vi "Save Raw Data.vi"(1 "data":T1[](array[typedef]) {"time (global)" format="%<%H:%M:%S\n%d/%m/%Y>T"}, 3 "time [ms]":i64, 7 "VI-data Save":T5={"Dateipfad save data"=path "", "file ref"=refnum, "number"=0, "Period [s]"=240, "Fehler (Ausgang)"={"status"=FALSE, "code"=0, "source"=""}}) -> (8 "VI-data Save out":T5={"Dateipfad save data"=path "", "file ref"=refnum, "number"=0, "Period [s]"=240, "Fehler (Ausgang)"={"status"=FALSE, "code"=0, "source"=""}})   [LabVIEW 2010, in "Licor-Steuerung.lvlib"]
uses:
  Licor-Steuerung.lvlib
  VI-data Save.ctl
  control/Licor-Parameter.ctl
  LicorLI7000/conventions/Licor-Source.ctl
  control/Licor-Pump.ctl
  LicorLI7000/conventions/output line.ctl
  LicorLI7000/LicorLI7000.lvlib
panel:
  in  "Licor-parameter":T2={"CO2 ref"=392.0, "CO2 span"=402.0, "H2O ref"=0.0, "H2O span"=0.0, "Zi"=1.2, "Zt"=0.0, "Zm"=0.0, "S"=1.0, "Temp [C]"=50.0, "Pressure [hPa]"=135.0, "Licor-Sources"=["CO2A W", "CO2B W", "H2OA W", "H2OB W", "T C", "T V", "P kPa", "P V", "RH %", "CO2A um/m", "CO2B um/m", "H2OA mm/m", "H2OB mm/m"], "Licor-Pump"="Off", "Zeitstempel"=timestamp(0 s since 1904-01-01)} {"Pressure [hPa]" format="%_5g"; "Temp [C]" format="%.2f"; "CO2 ref" format="%.2f"; "CO2 span" format="%.2g"; "H2O ref" format="%.2g"; "H2O span" format="%.2g"; "Zt" format="%#_4g"}
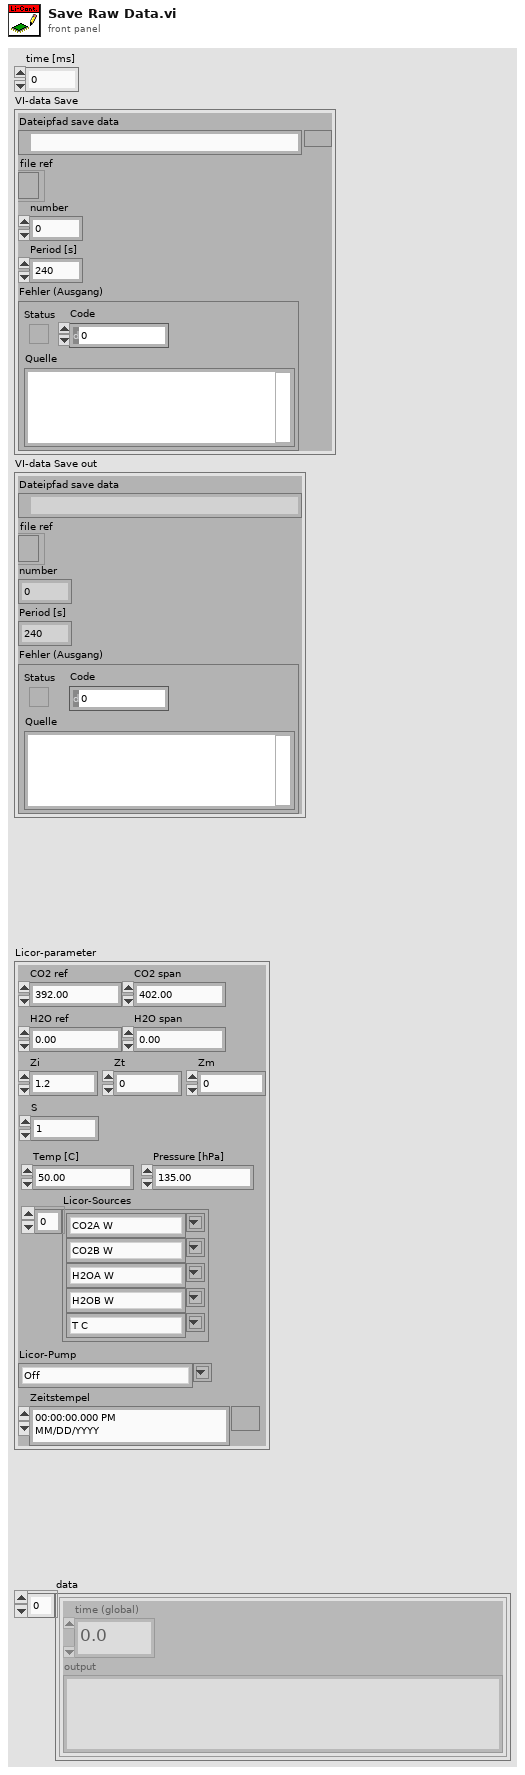
[diagram p1: front panel]
types:
  T1 = typedef "LicorLI7000.lvlib/output line.ctl" = cluster{"time (global)":dbl, "output":string}
  T2 = typedef "Licor-Steuerung.lvlib/Licor-Parameter.ctl" = cluster{"CO2 ref":dbl, "CO2 span":dbl, "H2O ref":dbl, "H2O span":dbl, "Zi":dbl, "Zt":dbl, "Zm":dbl, "S":dbl, "Temp [C]":dbl, "Pressure [hPa]":dbl, "Licor-Sources":T3[], "Licor-Pump":T4, "Zeitstempel":timestamp}
  T3 = typedef "LicorLI7000.lvlib/Licor-Source.ctl" = string
  T4 = typedef "Licor-Steuerung.lvlib/Licor-Pump.ctl" = string
  T5 = typedef "Licor-Steuerung.lvlib/VI-data Save.ctl" = cluster{"Dateipfad save data":path, "file ref":refnum<file>, "number":i64, "Period [s]":i64, "Fehler (Ausgang)":errorcluster}
  T6 = enum16{"open", "replace", "create", "open or create", "replace or create", "replace or create with confirmation"}
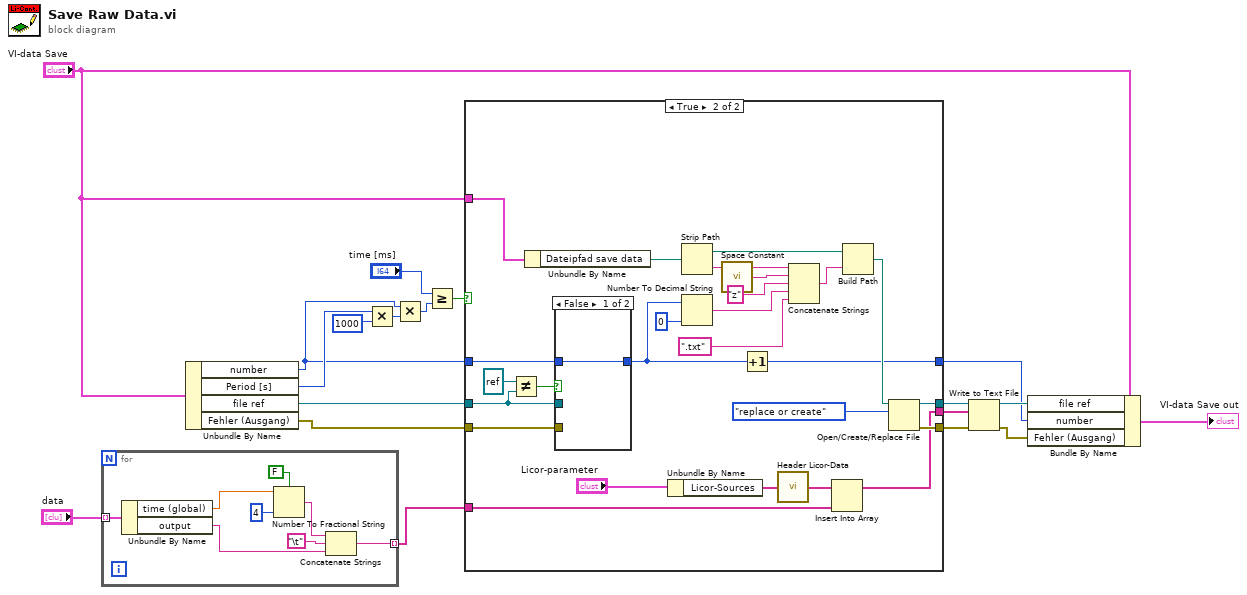
[diagram p0: block diagram]
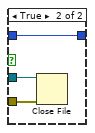
[diagram p3: hidden frame]
diagram:
  n1 = for {
    tunnel: "data" -> [w27] mode=indexing
    tunnel: [w20] -> w1 mode=indexing
    n2 = Unbundle By Name(w27) -> ("time (global)"=w26:dbl, "output"=w25:string)
    n3 = Number To Fractional String(use system decimal point (T)=FALSE ("Systemdezimalzeichen verwenden (T)"), number=w26, precision (6)=i16 4 ("Genauigkeit (6)")) -> (F-format string=w24:string)  [unwired: 1 in]
    n4 = Concatenate Strings(w24, "\t", w25) -> (w20:string)
  }
  n5 = Unbundle By Name("VI-data Save") -> ("number"=w3:i64, "Period [s]"=w4:i64, "file ref"=w5:refnum<file>, "Fehler (Ausgang)"=w7:errorcluster)
  n6 = Multiply(x=w4, y=i64 1000) -> (x*y=w12:i64)
  n7 = Multiply(x=w3, y=w12) -> (x*y=w18:i64)
  n8 = Greater Or Equal?(x="time [ms]", y=w18) -> (x >= y?=w19:bool)
  n9 = case shown="True" w19 {
    tunnel: [w31 w32] -> w8
    tunnel: w3 -> [w31 w47]
    tunnel: [w30 w46] -> w16
    tunnel: w5 -> [w30 w48]
    tunnel: [w29 w55] -> w17
    tunnel: w7 -> [w29 w57]
    tunnel: w1 -> [w28 w52]
    tunnel: [w28 w51] -> w14
    tunnel: "VI-data Save" -> [_ w36]
    frame False {
    }
    frame True {
      n10 = Not Equal?(x=refnum<file> refnum ("y"), y=w48) -> (x != y?=w50:bool)
      n11 = Unbundle By Name(w36) -> ("Dateipfad save data"=w35:path)
      n12 = case shown="False" w50 {
        tunnel: w57 -> [_ w61]
        tunnel: w48 -> [_ w60]
        tunnel: w47 -> [w58 w59]
        tunnel: [w58 w59] -> w33
        frame False {
        }
        frame True {
          n13 = Close File(refnum=w60, error in=w61) -> ()  [unwired: 2 out]
        }
      }
      n14 = Unbundle By Name("Licor-parameter") -> ("Licor-Sources"=w54:T3[])
      n15 = Strip Path(path=w35) -> (stripped path=w45:path, name=w44:string)
      n16 = Number To Decimal String(number=w33, width (-)=i16 0 ("Breite (-)")) -> (decimal integer string=w40:string)
      n17 = call <vilib>:"Space Constant.vi"() -> ("String"=w42:string)
      n18 = Increment(x=w33) -> (x+1=w32:i64)
      n19 = call "Header Licor-Data.vi"("Licor-Sources"=w54) -> ("Header"=w53:string[])  [unwired: 14 in]
      n20 = Concatenate Strings(w44, w42, "z", w40, ".txt") -> (w38:string)
      n21 = Insert Into Array(array=w53, new element=w52) -> (w51:string[])  [unwired: 1 in]
      n22 = Build Path(base path=w45, name or relative path=w38) -> (appended path=w37:path)
      n23 = Open/Create/Replace File(file path (use dialog)=w37, operation (0:open)=T6."replace or create" ("Operation (0:Öffnen)")) -> (refnum out=w46:refnum<file>, error out=w55:errorcluster)  [unwired: 4 in, 1 out]
    }
  }
  n24 = Write to Text File(file (use dialog)=w16, text=w14, error in=w17) -> (refnum out=w10:refnum<file>, error out=w9:errorcluster)  [unwired: 1 in, 1 out]
  n25 = Bundle By Name(cluster="VI-data Save", "file ref"=w10, "number"=w8, "Fehler (Ausgang)"=w9) -> (→"VI-data Save out":T5)
